vi "GFITS_LibWriteFromBuf.vi"(8 "error in (no error)":errorcluster, 9 "eleRead":i32, 10 "amplifiers":u64, 11 "fd":u64) -> (0 "error out":errorcluster, 1 "progress out":i32, 2 "return value":i32, 3 "fd out":u64, 4 "zcnt out":i32, 7 "num_amps":i32)   [LabVIEW 2016]
uses:
  c/lib/libgfits.so
panel:
  in  "num_amps in":i32
  in  "zcnt in":i32
  in  "progress in":i32
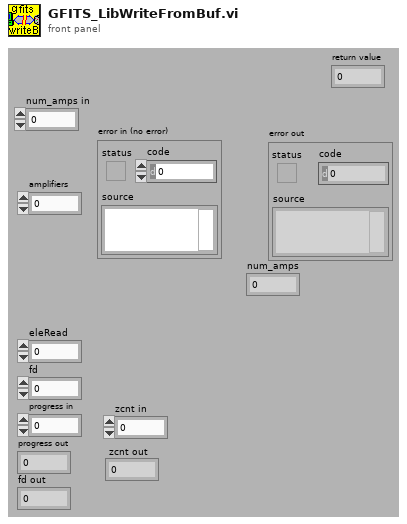
[diagram p1: front panel]
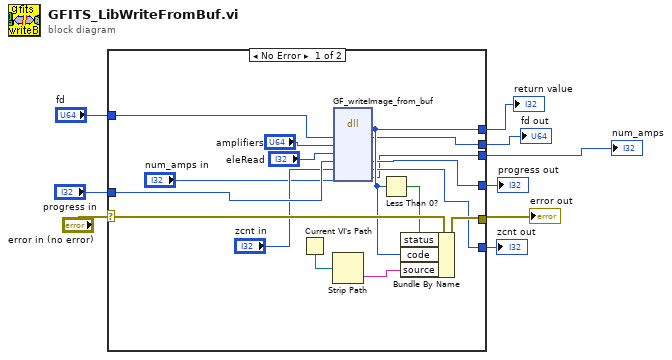
[diagram p0: block diagram]
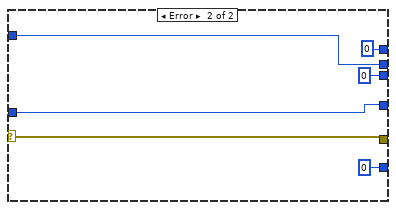
[diagram p2: hidden frame]
diagram:
  n1 = case shown="No Error" "error in (no error)" {
    selector: "error in (no error)" -> [w25 w31]
    tunnel: [w23 0] -> w9
    tunnel: [w20 w31] -> w7
    tunnel: [w17 w29] -> w6
    tunnel: "progress in" -> [w16 w29]
    tunnel: "fd" -> [w15 w28]
    tunnel: [w14 w28] -> w3
    tunnel: [w12 0 ("zcnt")] -> w2
    tunnel: [w10 0 ("num_amps")] -> w1
    frame No Error {
      n2 = Current VI's Path() -> (path=w22:path)
      n3 = Strip Path(path=w22) -> (name=w21:string)  [unwired: 1 out]
      n4 = dll-call lib="home/simager/panview/PAN/Modules/GFITS/private/c/lib/libgfits.so" fn="GF_writeImage_from_buf"("fd"=w15, "buffer"="amplifiers", "eleRead"="eleRead", "progress"=w16, "zcnt"="zcnt in", "num_amps"="num_amps in") -> ("return type"=w23:i32, "fd"=w14:u64, "progress"=w17:i32, "zcnt"=w12:i32, "num_amps"=w10:i32)  [unwired: 5 in, 2 out]
      n5 = Less Than 0?(x=w23) -> (x < 0?=w24:bool)
      n6 = Bundle By Name(cluster=w25, "status"=w24, "code"=w23, "source"=w21) -> (w20:errorcluster)
    }
    frame Error {
    }
  }
  "return value" <- w9
  "error out" <- w7
  "progress out" <- w6
  "fd out" <- w3
  "zcnt out" <- w2
  "num_amps" <- w1
